vi "Part_GetAttributes.vi"(0 "reference in":refnum<class "Part.lvclass">, 1 "return data? (T)":bool=TRUE, 5 "error in (no error)":errorcluster) -> (14 "reference out":refnum<class "Part.lvclass">, 15 "attributes ref":T2, 16 "attributes":T1, 19 "error out":errorcluster)   [LabVIEW 2013, in "Part.lvclass"]
doc: "Returns a reference and if wanted the actual data values of the attributes. This method is used by the subclasses to access parent attributes."
uses:
  Part.lvclass
  ObjectAttributesRef.ctl
  protected/ObjectAttributes.ctl
  Part.lvclass/Part.ctl
  <vilib>/addons/_AddQ/G#Object/G#Object.lvclass
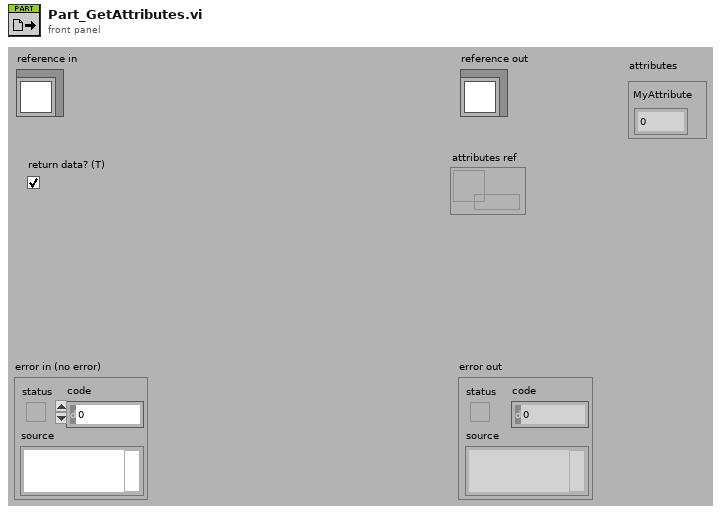
[diagram p1: front panel]
types:
  T1 = typedef "Part.lvclass/ObjectAttributes.ctl" = cluster{"MyAttribute":dbl}
  T2 = typedef "Part.lvclass/ObjectAttributesRef.ctl" = refnum<data-value>
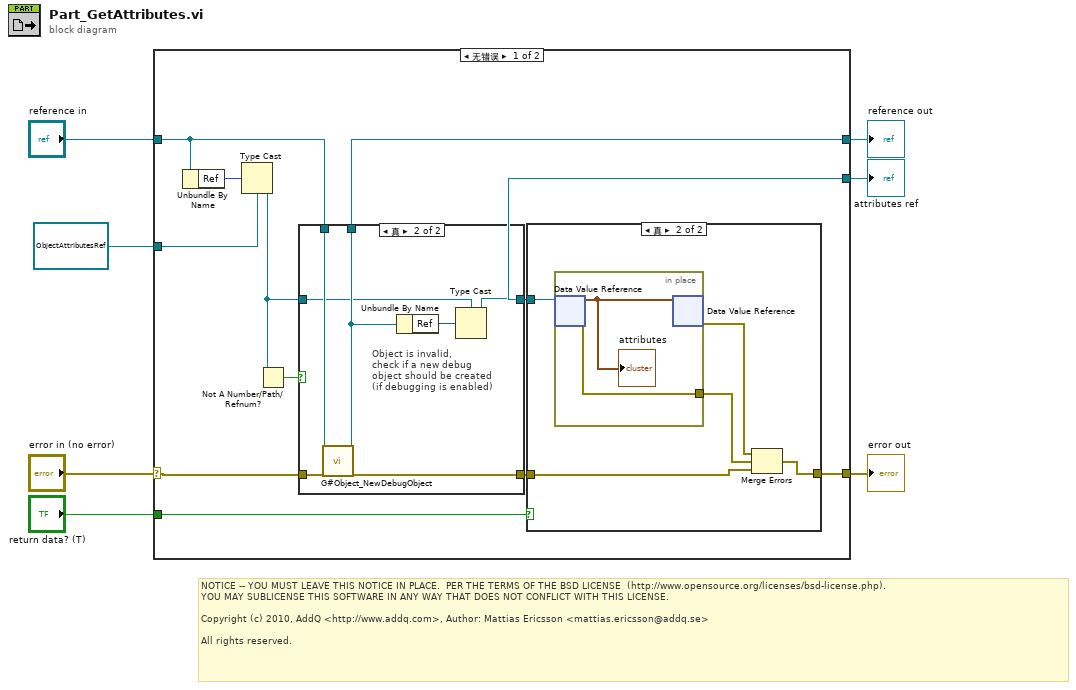
[diagram p0: block diagram]
diagram:
  # "NOTICE -- YOU MUST LEAVE THIS NOTICE IN PLACE.  PER THE TERMS OF THE BSD LICENSE  (http://www.opensource.org/licenses/bsd-license.php).\nYOU MAY SUBLICENSE THIS SOFTWARE IN ANY WAY THAT DOES NOT CONFLICT WITH THIS LICENSE.\n\nCopyright (c) 2010, AddQ <http://www.addq.com>, Author: Mattias Ericsson <mattias.ericsson@addq.se>\n\nAll rights reserved."
  n1 = case shown="无错误" "error in (no error)" {
    selector: "error in (no error)" -> [w14 w39]
    tunnel: [w17 w39] -> w6
    tunnel: [w11 w38] -> w4
    tunnel: "reference in" -> [w12 w38]
    tunnel: [w8 w37] -> w3
    tunnel: "return data? (T)" -> [w18 _]
    tunnel: T2 refnum ("attributes ref") -> [w10 w37]
    frame No Error {
      n2 = Unbundle By Name(w12) -> ("Ref"=w16:u32)
      n3 = Type Cast(type=w10, x=w16) -> (*(type *) &x=w9:T2)
      n4 = Not A Number/Path/Refnum?(number/path/refnum=w9) -> (NaN/Path/Refnum?=w13:bool)
      n5 = case shown="真" w13 {
        tunnel: [w21 w28] -> w15
        tunnel: w14 -> [w21 w27]
        tunnel: w12 -> [w20 w26]
        tunnel: [w20 w24] -> w11
        tunnel: w9 -> [w19 w23]
        tunnel: [w19 w22] -> w8
        frame False {
        }
        frame True {
          # "Object is invalid,\ncheck if a new debug\nobject should be created\n(if debugging is enabled)"
          n6 = call <vilib>:"G#Object_NewDebugObject.vi"("reference in"=w26, "error in (no error)"=w27) -> ("reference out"=w24:refnum<class "Part.lvclass">, "error out"=w28:errorcluster)  [unwired: 16 in]
          n7 = Unbundle By Name(w24) -> ("Ref"=w25:u32)
          n8 = Type Cast(type=w23, x=w25) -> (*(type *) &x=w22:T2)
        }
      }
      n9 = case shown="真" w18 {
        tunnel: w8 -> [_ w34]
        tunnel: w15 -> [w29 w33]
        tunnel: [w29 w30] -> w17
        frame False {
        }
        frame True {
          n10 = in-place {
            in-place-border: [w36] -> w32
            n11 = in-place-dvr #1(w34) -> (w35:T1, w36:errorcluster)
            "attributes" <- w35
            n12 = in-place-dvr #1(w35) -> (w31:errorcluster)  [unwired: 1 out]
          }
          n13 = Merge Errors(w31, w32, w33) -> (w30:errorcluster)
        }
      }
    }
    frame Error {
    }
  }
  "error out" <- w6
  "reference out" <- w4
  "attributes ref" <- w3
